vi "Line Configuration Dialog.vi"(8 "error in":errorcluster, 9 "engine configuration in":refnum<class "engine configuration.lvclass">, 10 "tag bus configurable plugin module configuration":refnum<class "J1939 configuration.lvclass">, 11 "Line":T4={"channel"=refnum, "XNET Signal"="CANEventSignal1\nNIXNET_example.CAN_Cluster"}) -> (0 "error out":errorcluster, 1 "success":bool, 2 "changed":bool, 3 "Mappings out":T3={"Line"={"channel"=refnum, "XNET Signal"="CANEventSignal1\nNIXNET_example.CAN_Cluster"}, "Maps"=[]})   [LabVIEW 2013, in "J1939 editor node.lvclass"]
doc: "A dialog for allowing a user to specify the values of a new line."
uses:
  J1939 editor node.lvclass
  module/configuration/Line.ctl
  <vilib>/NI/Tag Bus Module Framework/channel/TBM channel.lvclass
  Mappings.ctl
  Map.ctl
  permissions.ctl
  <vilib>/NI/Module Execution Interface/Engine Configuration/engine configuration.lvclass
  module/configuration/J1939 configuration.lvclass
  <vilib>/NI/Tag Bus/tag/Data Type.ctl
  <vilib>/NI/Tag Bus Module Framework/channel/TBM channel.lvclass/TBM channel.ctl
  <vilib>/NI/Configuration Framework/serializable configuration/NISE_CEF_serializable configuration.lvclass/NISE_CEF_serializable configuration.ctl
  <vilib>/NI/Tag Bus Module Framework/channel/channel classification.ctl
  <vilib>/NI/Tag Bus/tag/tag descriptor.lvclass/tag descriptor.ctl
  <vilib>/NI/Tag Bus/tag/write tag name.vi
  <vilib>/NI/Tag Bus/tag/write data type.vi
  <vilib>/NI/Tag Bus Module Framework/channel/Write channel classification.vi
  <vilib>/NI/Configuration Framework/serializable configuration/Read UID.vi
  <vilib>/NI/Tag Bus Module Framework/channel/Read channel classification.vi
  <vilib>/Utility/LVClass/Get LV Class Name.vi
  <vilib>/NI/Configuration Framework/error generator/NISE_error generator.vi
  <vilib>/NI/Tag Bus/tag/tag descriptor.lvclass
  <vilib>/NI/DCAF UI Toolkit/Controls/DCAF UI Elements.lvlib
panel:
  out "Data Type":T1
  in  "XNET Signal":refnum<k21>="CANEventSignal1\nNIXNET_example.CAN_Cluster"
  out "errors":string
  in  "Access Type":T2
  in  "Tag":i32(listbox)
  in  "cancel":bool
  in  "ok":bool
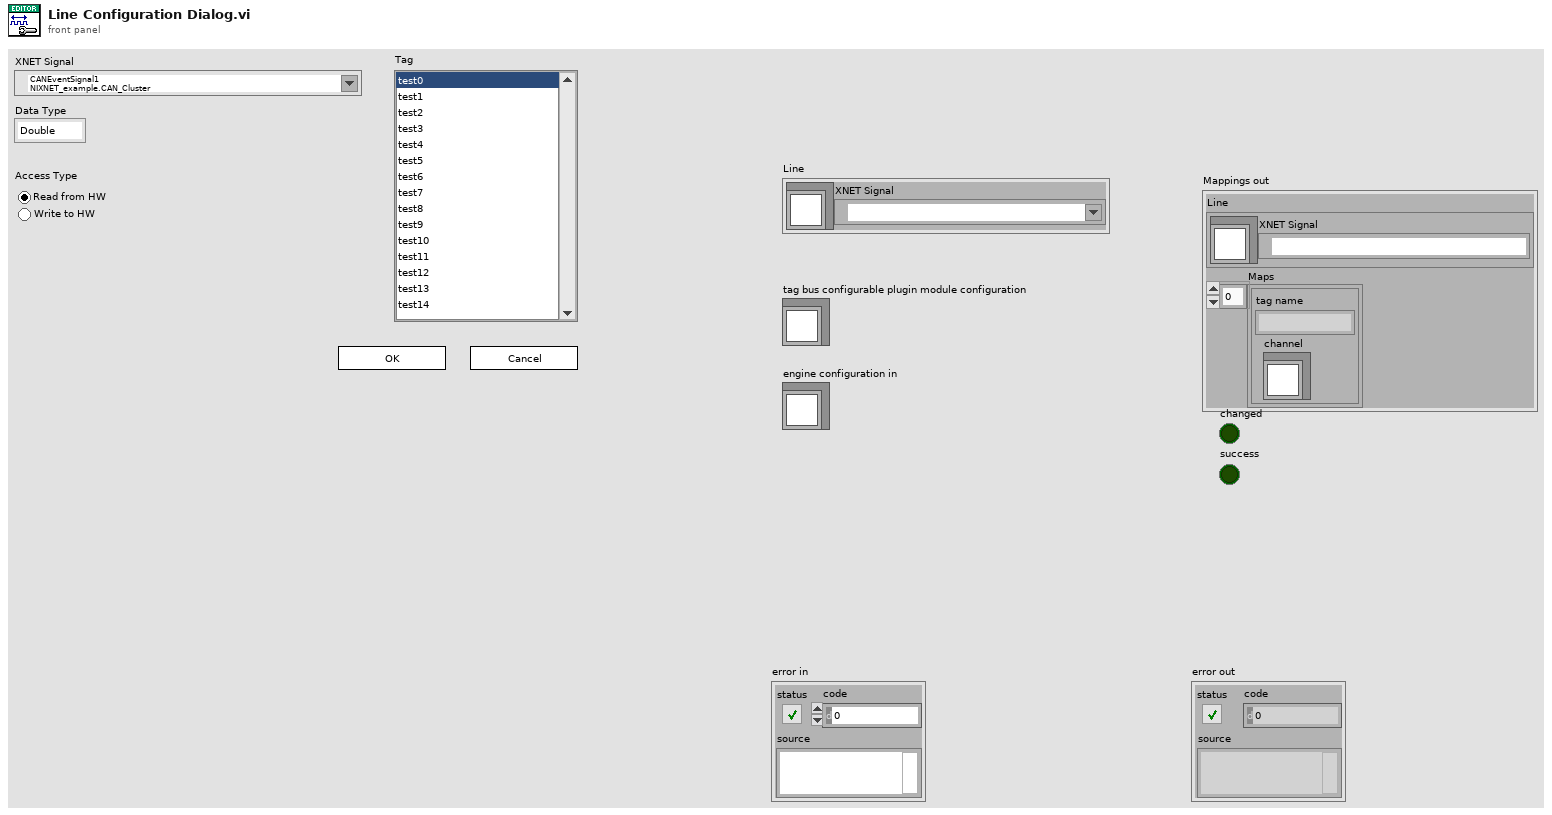
[diagram p1: front panel]
types:
  T1 = typedef "tag bus.lvlib/tag descriptor.lvclass/Data Type.ctl" = enum16{"Double", "Single", "I64", "I32", "I16", "I8", "U64", "U32", "U16", "U8", "Boolean", "String", "Array of Double", "Array of Single", "Array of I64", "Array of I32", "Array of I16", "Array of I8", "Array of U64", "Array of U32", "Array of U16", "Array of U8", "Array of Boolean", "Array of String"}
  T2 = typedef "J1939 editor node.lvclass/permissions.ctl" = enum32{"Read from HW", "Write to HW"}
  T3 = typedef "J1939 editor node.lvclass/Mappings.ctl" = cluster{"Line":T4, "Maps":T5[]}
  T4 = typedef "J1939 configuration.lvclass/Line.ctl" = cluster{"channel":refnum<class "TBM channel.lvclass">, "XNET Signal":refnum<k21>}
  T5 = typedef "J1939 editor node.lvclass/Map.ctl" = cluster{"channel":refnum<class "TBM channel.lvclass">, "tag name":string}
  T6 = typedef "TBM channel.lvclass/channel classification.ctl" = enum16{"input data", "output data", "processing parameter", "processing result"}
  T7 = enum8{"Enabled", "Disabled", "Disabled and Grayed Out"}
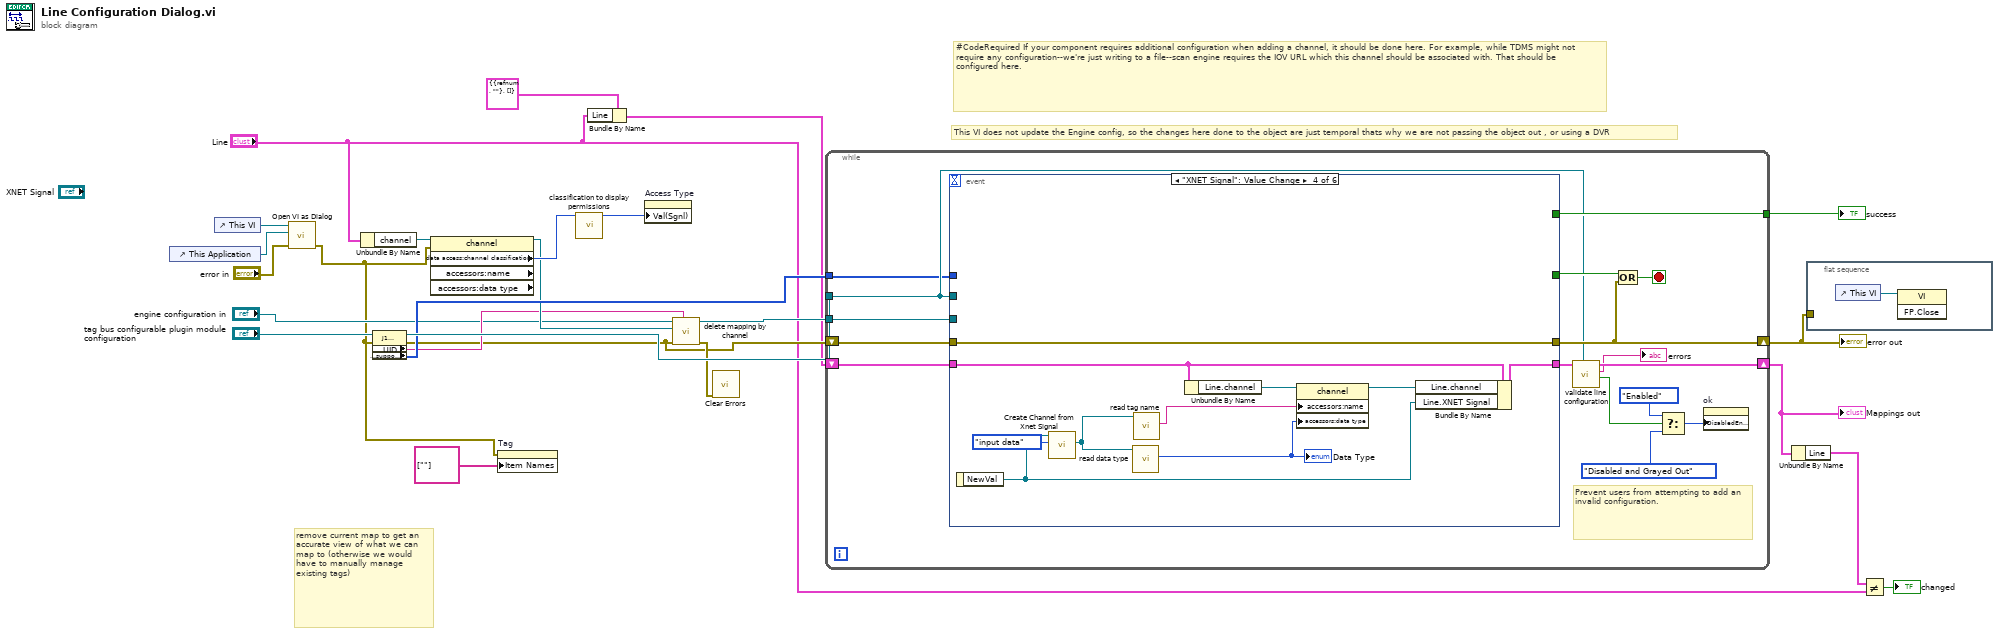
[diagram p0: block diagram]
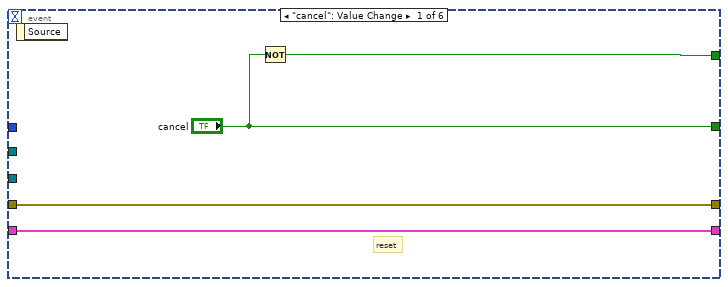
[diagram p2: hidden frame]
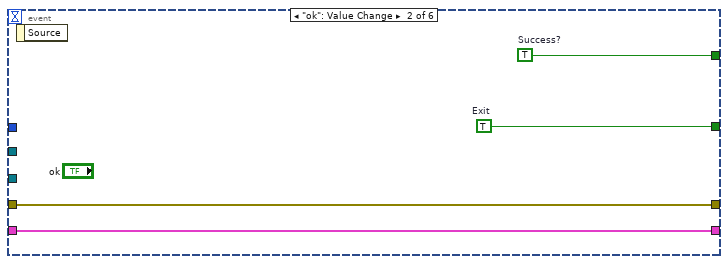
[diagram p3: hidden frame]
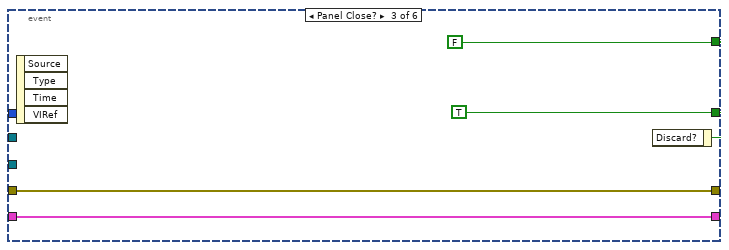
[diagram p4: hidden frame]
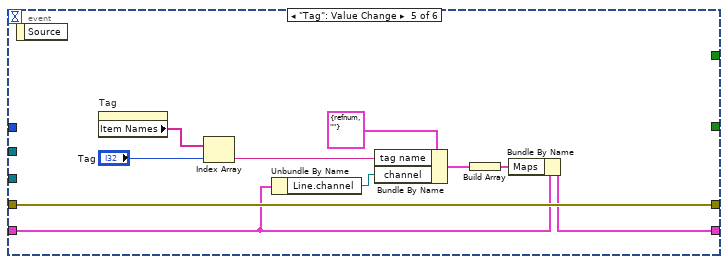
[diagram p5: hidden frame]
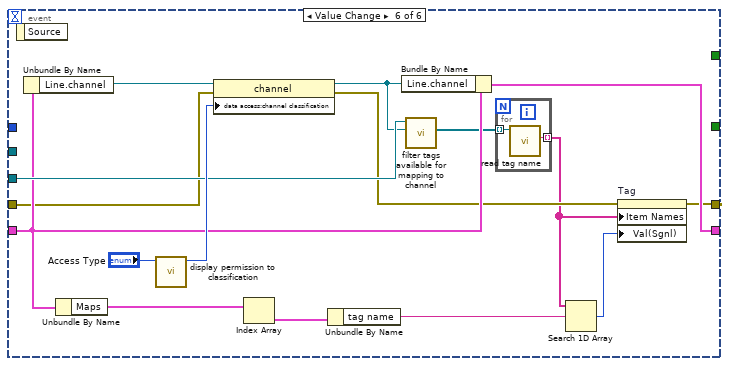
[diagram p6: hidden frame]
diagram:
  # "This VI does not update the Engine config, so the changes here done to the object are just temporal thats why we are not passing the object out , or using a DVR"
  # "remove current map to get an accurate view of what we can map to (otherwise we would have to manually manage existing tags)"
  # "#CodeRequired If your component requires additional configuration when adding a channel, it should be done here. For example, while TDMS might not require any configuration--we're just writing to a file--scan engine requires the IOV URL which this channel should be associated with. That should be configured here."
  n1 = control-ref of="This Application"() -> (w3:refnum<vi>)
  n2 = control-ref of="This VI"() -> (w4:refnum<vi>)
  n3 = call <vilib>:"Open VI as Dialog.vi"("error in (no error)"="error in", "This Application"=w3, "VI in"=w4) -> ("error out"=w1:errorcluster)  [unwired: 8 in]
  n4 = Unbundle By Name("Line") -> ("channel"=w18:refnum<class "TBM channel.lvclass">)
  n5 = property class="J1939 configuration"(reference="tag bus configurable plugin module configuration", error in=w1) -> (reference out=w22:refnum<class "J1939 configuration.lvclass">, error out=w11:errorcluster, "Properties:UID"=w16:string, "Customize:Properties:supported types"=w21:T1[])
  n6 = property class="channel" props=["data access:channel classification", "accessors:name", "accessors:data type"](reference=w18, error in=w1) -> (reference out=w17:refnum<class "TBM channel.lvclass">, "data access:channel classification"=w19:T6)  [unwired: 3 out]
  n7 = property on="Tag" class="LstBox (strict)"(error in=w1, "Item Names"=string[] [""]) -> ()  [unwired: 1 in, 2 out]
  n8 = call "classification to display permissions.vi"("channel classification"=w19) -> ("permissions"=w14:T2)  [unwired: 10 in]
  n9 = Bundle By Name(cluster=T3 {"Line"={"channel"=refnum, "XNET Signal"=""}, "Maps"=[]} ("Mappings out"), "Line"="Line") -> (w7:T3)
  n10 = property on="Access Type" class="RadioBtnsControl (strict)"("Val(Sgnl)"=w14) -> ()  [unwired: 2 in, 2 out]
  n11 = call <vilib>:"delete mapping by channel.vi"("owner ID"=w16, "error in"=w11, "channel"=w17, "engine configuration in"="engine configuration in") -> ("error out"=w13:errorcluster, "engine configuration out"=w23:refnum<class "engine configuration.lvclass">)  [unwired: 6 in]
  n12 = call <vilib>:"Clear Errors.vi"("error in (no error)"=w13) -> ()  [unwired: 6 in, 1 out]
  n13 = while {
    shift-right: [w33] -> w20
    shift-left: w11 -> [w40]
    tunnel: [w39] -> w25
    shift-right: [w34] -> w5
    shift-left: w7 -> [w36]
    tunnel: w23 -> [w41]
    tunnel: w22 -> [w28]
    tunnel: w21 -> [w27]
    stop <- w37 stop-if-true
    # "Prevent users from attempting to add an invalid configuration."
    n14 = event shown="[3] \"XNET Signal\": Value Change" {
      selector: _ -> [_ _ _ _ _ _]
      dyn-events: _ -> [_ _ _ _ _ _]
      timeout: _ -> [_ _ _ _ _ _]
      tunnel: w41 -> [_ _ _ _ _ w87]
      tunnel: w40 -> [w45 w49 w53 w63 w73 w81]
      tunnel: [w45 w49 w53 w63 w73 w79] -> w33
      tunnel: [w44 w46 FALSE _ _ _] -> w39
      tunnel: ["cancel" w47 w51 _ _ _] -> w38
      tunnel: w36 -> [w42 w48 w50 w61 w67 w85]
      tunnel: [w42 w48 w50 w62 w64 w84] -> w35
      tunnel: w28 -> [_ _ _ _ _ _]
      tunnel: w27 -> [_ _ _ _ _ _]
      event "cancel": Value Change {
        # "reset"
        n15 = event-data() -> ()  [unwired: 1 in, 1 out]
        n16 = Not(x="cancel") -> (.not. x?=w44:bool)
      }
      event "ok": Value Change {
        w46 = TRUE  # Success?
        w47 = TRUE  # Exit
        n17 = event-data() -> ()  [unwired: 1 in, 1 out]
      }
      event Panel Close? {
        w51 = TRUE ("cancel")
        n18 = event-data() -> ()  [unwired: 1 in, 4 out]
        n19 = event-data("Discard?"=w51) -> ()  [unwired: 1 in, 1 out]
      }
      event "XNET Signal": Value Change {
        n20 = event-data() -> ("NewVal"=w58:refnum<k21>)  [unwired: 1 in]
        n21 = call "Create Channel from Xnet Signal.vi"("channel classification"=channel_classification."input data", "XNET Signal"=w58) -> ("channel"=w56:refnum<class "TBM channel.lvclass">)  [unwired: 7 in, 2 out]
        n22 = call <vilib>:"read data type.vi"("system tag in"=w56) -> ("data type"=w54:T1)  [unwired: 8 in, 2 out]
        "Data Type" <- w54
        n23 = call <vilib>:"read tag name.vi"("system tag in"=w56) -> ("name"=w55:string)  [unwired: 8 in, 2 out]
        n24 = Unbundle By Name(w61) -> ("Line.channel"=w60:refnum<class "TBM channel.lvclass">)
        n25 = property class="channel"(reference=w60, "accessors:name"=w55, "accessors:data type"=w54) -> (reference out=w59:refnum<class "TBM channel.lvclass">)  [unwired: 1 in, 1 out]
        n26 = Bundle By Name(cluster=w61, "Line.channel"=w59, "Line.XNET Signal"=w58) -> (w62:T3)
      }
      event "Tag": Value Change {
        n27 = event-data() -> ()  [unwired: 1 in, 1 out]
        n28 = property on="Tag" class="LstBox (strict)"() -> ("Item Names"=w71:string[])  [unwired: 2 in, 2 out]
        n29 = Index Array(array=w71, index="Tag") -> (element=w70:string)
        n30 = Unbundle By Name(w67) -> ("Line.channel"=w68:refnum<class "TBM channel.lvclass">)
        n31 = Bundle By Name(cluster=T5 {"channel"=refnum, "tag name"=""} ("Map"), "tag name"=w70, "channel"=w68) -> (w66:T5)
        n32 = Build Array(w66) -> (w65:T5[])
        n33 = Bundle By Name(cluster=w67, "Maps"=w65) -> (w64:T3)
      }
      event Value Change {
        n34 = event-data() -> ()  [unwired: 1 in, 1 out]
        n35 = Unbundle By Name(w85) -> ("Line.channel"=w89:refnum<class "TBM channel.lvclass">)
        n36 = Unbundle By Name(w85) -> ("Maps"=w76:T5[])
        n37 = call "display permission to classification.vi"("display permissions"="Access Type") -> ("channel classification"=w88:T6)  [unwired: 10 in]
        n38 = property class="channel"(reference=w89, error in=w81, "data access:channel classification"=w88) -> (reference out=w86:refnum<class "TBM channel.lvclass">, error out=w80:errorcluster)
        n39 = Index Array(array=w76) -> (element=w75:T5)  [unwired: 1 in]
        n40 = Unbundle By Name(w75) -> ("tag name"=w74:string)
        n41 = Bundle By Name(cluster=w85, "Line.channel"=w86) -> (w84:T3)
        n42 = call <vilib>:"filter tags available for mapping to channel.vi"("channel to map to"=w86, "engine configuration in"=w87) -> ("filtered tags"=w83:refnum<class "tag descriptor.lvclass">[])  [unwired: 8 in, 1 out]
        n43 = for {
          tunnel: w83 -> [w91] mode=indexing
          tunnel: [w90] -> w78 mode=indexing
          n44 = call <vilib>:"read tag name.vi"("system tag in"=w91) -> ("name"=w90:string)  [unwired: 8 in, 2 out]
        }
        n45 = Search 1D Array(1D array=w78, element=w74) -> (index of element=w77:i32)  [unwired: 1 in]
        n46 = property on="Tag" class="LstBox (strict)"(error in=w80, "Item Names"=w78, "Val(Sgnl)"=w77) -> (error out=w79:errorcluster)  [unwired: 1 in, 1 out]
      }
    }
    n47 = call "validate line configuration.vi"("Module Config"=w28, "Mappings in"=w35) -> ("valid?"=w32:bool, "errors"=→"errors":string, "Mappings out"=w34:T3)  [unwired: 7 in]
    n48 = Compound Arithmetic op=OR(w38, w33) -> (w37:bool)
    n49 = Select(t=T7."Enabled" ("Disabled"), s=w32, f=T7."Disabled and Grayed Out") -> (s? t:f=w29:T7)
    n50 = property on="ok" class="Bool"("DisabledEnum"=w29) -> ()  [unwired: 2 in, 2 out]
  }
  "error out" <- w20
  "success" <- w25
  "Mappings out" <- w5
  n51 = Unbundle By Name(w5) -> ("Line"=w6:T4)
  n52 = flat-sequence {
    tunnel: w20 -> [_]
    frame #0 {
      n53 = control-ref of="This VI"() -> (w92:refnum<vi>)
      n54 = invoke class="VI" method="FP.Close"(reference=w92) -> ()  [unwired: 2 in, 3 out]
    }
  }
  n55 = Not Equal?(x=w6, y="Line") -> (x != y?=→"changed":bool)
